vi "close ASI stage.vi"(8 "error in (no error)":errorcluster, 11 "ASI stage":T1) -> (0 "error out":errorcluster, 3 "ASI stage out":T1)   [LabVIEW 2010]
uses:
  stage properties.ctl
  <vilib>/Instr/_visa.llb/VISA Flush IO Buffer Mask.ctl
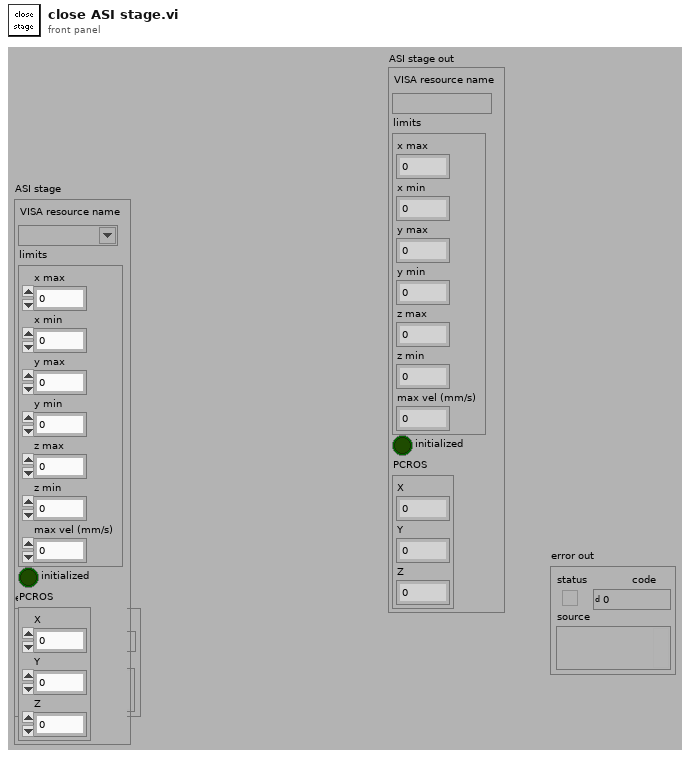
[diagram p1: front panel]
types:
  T1 = typedef "stage properties.ctl" = cluster{"VISA resource name":refnum<visa-resource-name>, "limits":cluster{"x max":dbl, "x min":dbl, "y max":dbl, "y min":dbl, "z max":dbl, "z min":dbl, "max vel (mm/s)":dbl}, "initialized":bool, "PCROS":cluster{"X":dbl, "Y":dbl, "Z":dbl}}
  T2 = typedef "VISA Flush IO Buffer Mask.ctl" = u16
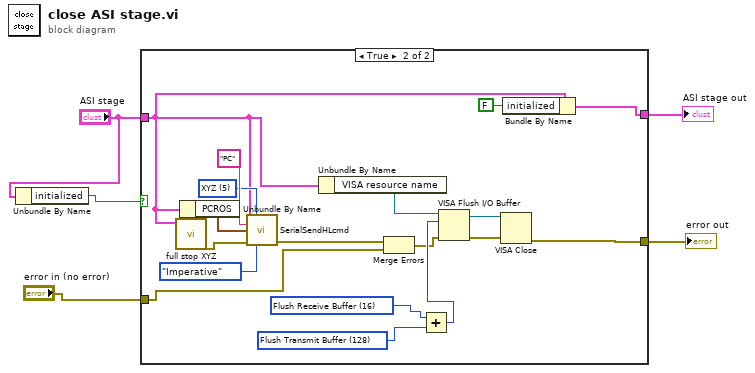
[diagram p0: block diagram]
diagram:
  n1 = Unbundle By Name("ASI stage") -> ("initialized"=w1:bool)
  n2 = case shown="True" w1 {
    tunnel: [w6 w19] -> w5
    tunnel: "ASI stage" -> [w7 w9]
    tunnel: [w7 w16] -> w4
    tunnel: "error in (no error)" -> [w6 w15]
    frame False {
    }
    frame True {
      w11 = u16 5 items=["No axis", "X", "Y", "Z", "XY", "XYZ"] ("Axis configuration")
      w25 = T2 128 items=["Flush Receive Buffer"=16, "Write Transmit Buffer to Device"=32, "Flush Receive Buffer (No I/O)"=64, "Flush Transmit Buffer"=128] ("Mask")
      w24 = T2 16 items=["Flush Receive Buffer"=16, "Write Transmit Buffer to Device"=32, "Flush Receive Buffer (No I/O)"=64, "Flush Transmit Buffer"=128] ("Mask")
      n3 = call "full stop XYZ.vi"("ASI stage"=w9) -> ("error out"=w14:errorcluster)  [unwired: 10 in]
      n4 = Unbundle By Name(w9) -> ("PCROS"=w8:cluster{"X":dbl, "Y":dbl, "Z":dbl})
      n5 = call "SerialSendHLcmd.vi"("ASI stage"=w9, "Axis configuration"=w11, "Command"="PC", "data in"=w8, "error in (no error)"=w14, "Command type"=enum16{"Query", "Where", "Imperative", "DU Y"}."Imperative") -> ("error out"=w13:errorcluster)  [unwired: 7 in, 2 out]
      n6 = Unbundle By Name(w9) -> ("VISA resource name"=w22:refnum<visa-resource-name>)
      n7 = Merge Errors(w13, w15) -> (w18:errorcluster)
      n8 = Add(x=w24, y=w25) -> (x+y=w23:T2)
      n9 = VISA Flush I/O Buffer(VISA resource name=w22, mask (16)=w23, error in (no error)=w18) -> (VISA resource name out=w20:refnum<visa-resource-name>, error out=w21:errorcluster)
      n10 = VISA Close(VISA resource name=w20, error in (no error)=w21) -> (error out=w19:errorcluster)
      n11 = Bundle By Name(cluster=w9, "initialized"=FALSE) -> (w16:T1)
    }
  }
  "error out" <- w5
  "ASI stage out" <- w4
